vi "Execute_Light Bathe.vi"(0 "VISA Refnum in":refnum<visa-resource-name>, 1 "Execute?":bool, 2 "Duration":dbl, 3 "error in (no error)":errorcluster) -> (7 "VISA Out":refnum<visa-resource-name>, 10 "Error Out":errorcluster)   [LabVIEW 2012]
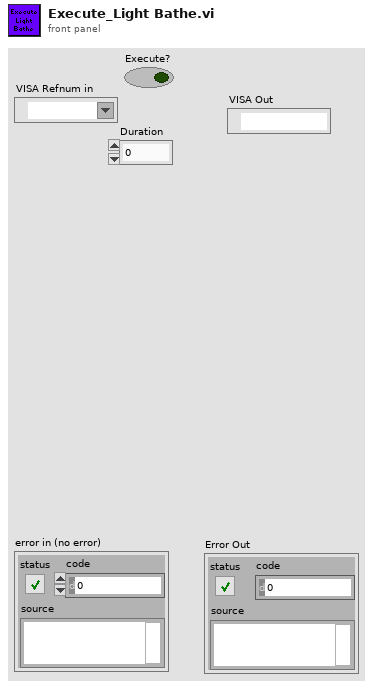
[diagram p1: front panel]
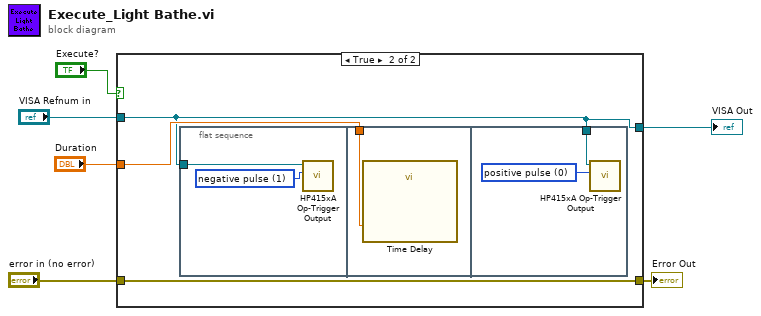
[diagram p0: block diagram]
diagram:
  n1 = case shown="True" "Execute?" {
    tunnel: "Duration" -> [_ w11]
    tunnel: "VISA Refnum in" -> [w7 w9]
    tunnel: "error in (no error)" -> [w8 w10]
    tunnel: [w8 w10] -> w2
    tunnel: [w7 w9] -> w1
    frame False {
    }
    frame True {
      n2 = flat-sequence {
        tunnel: w9 -> [w12]
        tunnel: w11 -> [w14]
        tunnel: w9 -> [w15]
        frame #0 {
          w13 = u32 1 items=["positive pulse  ", "negative pulse  ", "level high  ", "level low  "] ("trigger signal")
          n3 = call "HP415xA Op-Trigger Output.vi"("trigger signal"=w13, "VISA session"=w12) -> ()  [unwired: 2 in, 1 out]
        }
        frame #1 {
          n4 = call "Time Delay"("Delay Time (s)"=w14) -> ()  [unwired: 10 in, 1 out]
        }
        frame #2 {
          w16 = u32 0 items=["positive pulse  ", "negative pulse  ", "level high  ", "level low  "] ("trigger signal")
          n5 = call "HP415xA Op-Trigger Output.vi"("trigger signal"=w16, "VISA session"=w15) -> ()  [unwired: 2 in, 1 out]
        }
      }
    }
  }
  "VISA Out" <- w1
  "Error Out" <- w2
